vi "solar Refnum Type Cast (To).vi"(1 "SOLAR":refnum<queue>) -> (0 "Refnum":T1)   [LabVIEW 2018]
doc: "This type casts to the solar reference."
uses:
  solar_ctl SOLAR Refnum.ctl
  solar_ctl SOLAR Global.ctl
  solar_ctl Target Global.ctl
  voyager/solar_voy_ctl Voyager Refnum.ctl
  qtimer/solar_qtimer_ctl Refnum.ctl
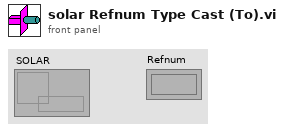
[diagram p1: front panel]
types:
  T1 = typedef "solar_ctl SOLAR Refnum.ctl" = refnum<k1>
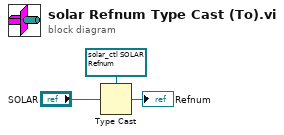
[diagram p0: block diagram]
diagram:
  w3 = T1 refnum items=["solar"] ("Refnum")
  n1 = Type Cast(type=w3, x="SOLAR") -> (*(type *) &x=→"Refnum":T1)
